vi "dosimat876_load_command.vi"(2 "error in":errorcluster, 3 "Method":string="Fill", 4 "Dosimat Port In":refnum<visa-resource-name>="COM1") -> (0 "error out":errorcluster, 1 "Dosimat Port Out":refnum<visa-resource-name>="COM1")   [LabVIEW 2010]
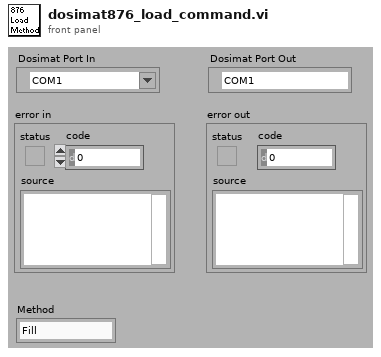
[diagram p1: front panel]
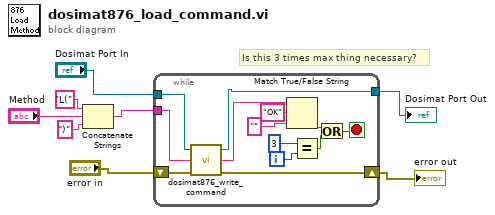
[diagram p0: block diagram]
diagram:
  # "Is this 3 times max thing necessary?"
  n1 = Concatenate Strings("L(" ("string"), "Method", ")" ("string")) -> (w8:string)
  n2 = while {
    tunnel: "Dosimat Port In" -> [w21]
    tunnel: w8 -> [w12]
    shift-right: [w11] -> w1
    shift-left: "error in" -> [w10]
    tunnel: [w9] -> w3
    i -> [w19]
    stop <- w17 stop-if-true
    n3 = call "dosimat876_write_command.vi"("error in"=w10, "write buffer"=w12, "Dosimat Port In"=w21) -> ("error out"=w11:errorcluster, "read buffer"=w20:string, "Dosimat Port Out"=w9:refnum<visa-resource-name>)
    n4 = Match True/False String(2:"" ("false string"), 3:"OK" ("true string"), 4:w20) -> (0:w16:bool)  [unwired: 1 out]
    n5 = Equal?(x=3, y=w19) -> (x = y?=w15:bool)
    n6 = Or(x=w16, y=w15) -> (x .or. y?=w17:bool)
  }
  "Dosimat Port Out" <- w3
  "error out" <- w1
